vi "test_Set Slot.vi"(8 "error in (no error)":errorcluster, 11 "TestCase in":refnum<class "Scan Engine Scripting API Custom Device Unit Tests.lvclass">) -> (0 "error out":errorcluster, 3 "TestCase out":refnum<class "Scan Engine Scripting API Custom Device Unit Tests.lvclass">)   [LabVIEW 2020, in "Scan Engine Scripting API Custom Device Unit Tests.lvclass"]
uses:
  Scan Engine Scripting API Custom Device Unit Tests.lvclass
  Scan Engine Scripting API Custom Device Unit Tests.lvclass/Scan Engine Scripting API Custom Device Unit Tests.ctl
  Scripting/Modules/NI 9475/NI 9475.lvclass
  <vilib>/Addons/_JKI Toolkits/VI Tester/TestCase.llb/TestCase.lvclass
  Scripting/Scan Engine Scripting.lvlib
  Scripting/Modules/Mode Classes/Controls/digital channel settings.ctl
  C:/Users/Administrator/Desktop/Jatin/All DNC DLLs/NationalInstruments.VeriStand.SystemDefinitionAPI.dll
  Jatin/All DNC DLLs/NationalInstruments.VeriStand.SystemDefinitionAPI.dll
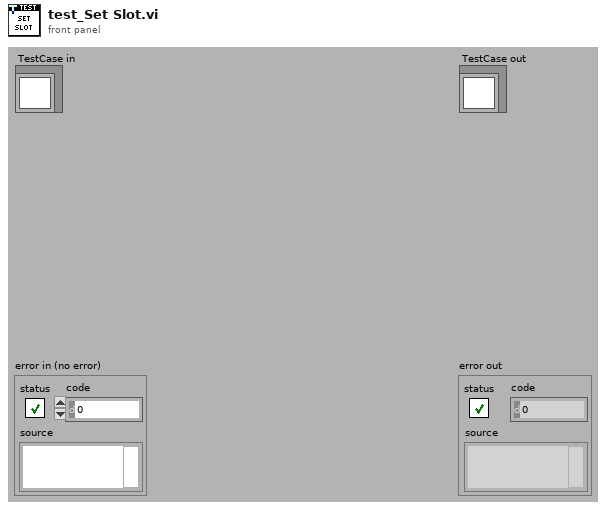
[diagram p1: front panel]
types:
  T1 = typedef "Scan Engine Scripting.lvlib/digital channel settings.ctl" = cluster{"name":string, "default value":bool}
  T2 = typedef "Custom Device API.lvlib/Custom Device Item Ref.ctl" = u64
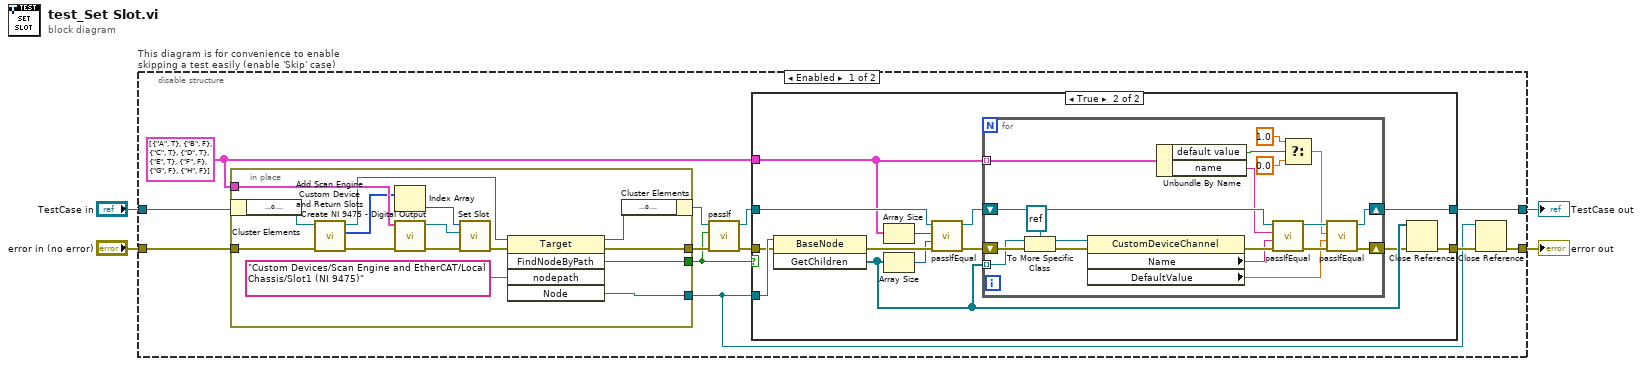
[diagram p0: block diagram]
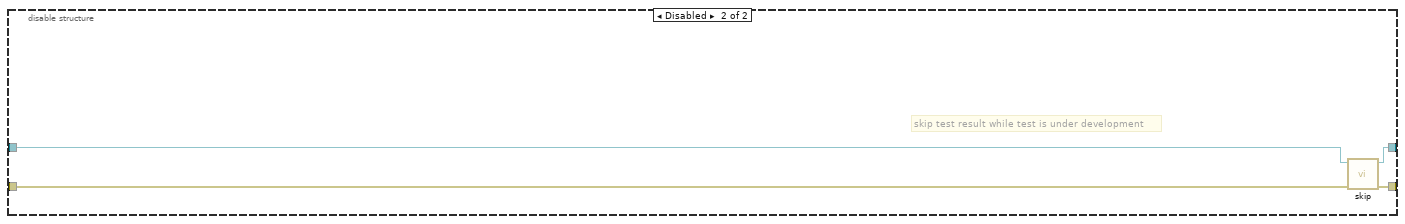
[diagram p3: hidden frame]
diagram:
  n1 = disable-structure "This diagram is for convenience to enable skipping a test easily (enable 'Skip' case)" shown="Enabled" {
    disable-tunnel: "TestCase in" -> [w8 w69]
    disable-tunnel: [w11 w67] -> w1
    disable-tunnel: [w10 w68] -> w3
    disable-tunnel: "error in (no error)" -> [w9 w66]
    frame Enabled {
      w6 = T1[] [{"name"="A", "default value"=TRUE}, {"name"="B", "default value"=FALSE}, {"name"="C", "default value"=TRUE}, {"name"="D", "default value"=TRUE}, {"name"="E", "default value"=TRUE}, {"name"="F", "default value"=FALSE}, {"name"="G", "default value"=FALSE}, {"name"="H", "default value"=FALSE}] ("channel settings")
      n2 = in-place {
        in-place-border: [w59] -> w16
        in-place-border: [w58] -> w5
        in-place-border: [w57] -> w15
        in-place-border: w9 -> [w55]
        in-place-border: w6 -> [w65]
        n3 = in-place-cluster #1(w8) -> ("target ref"=w52:refnum<k24>)
        n4 = call "Add Scan Engine Custom Device and Return Slots.vi"("error in"=w55, "NationalInstruments.VeriStand.SystemDefinitionAPI.Target"=w52) -> ("error out"=w54:errorcluster, "slot refs"=w53:T2[], "NationalInstruments.VeriStand.SystemDefinitionAPI.Target"=w56:refnum<k39>)  [unwired: 7 in]
        n5 = Index Array(array=w53) -> (element=w64:T2)  [unwired: 1 in]
        n6 = call "Create NI 9475 - Digital Output.vi"("error in"=w54, "channel settings"=w65) -> ("error out"=w63:errorcluster, "NI 9475 out"=w62:refnum<class "NI 9475.lvclass">)  [unwired: 8 in]
        n7 = call "Set Slot.vi"("error in"=w63, "module"=w62, "slot ref in"=w64) -> ("error out"=w61:errorcluster)  [unwired: 7 in, 1 out]
        n8 = invoke class="Target" method="FindNodeByPath"(reference=w56, error in=w61, "nodepath"="Custom Devices/Scan Engine and EtherCAT/Local Chassis/Slot1 (NI 9475)") -> (reference out=w51:refnum<k39>, error out=w59:errorcluster, "FindNodeByPath"=w57:bool, "Node"=w58:refnum<k39>)  [unwired: 2 in, 1 out]
        n9 = in-place-cluster #1("target ref"=w51) -> (w7:refnum<class "Scan Engine Scripting API Custom Device Unit Tests.lvclass">)
      }
      n10 = call-dynamic "passIf.vi"("error in (no error)"=w16, "pass"=w15, "TestCase in"=w7) -> ("error out"=w13:errorcluster, "TestCase out"=w14:refnum<class "Scan Engine Scripting API Custom Device Unit Tests.lvclass">)  [unwired: 7 in]
      n11 = case shown="True" w15 {
        tunnel: w13 -> [w17 w30]
        tunnel: w14 -> [w18 w29]
        tunnel: w5 -> [_ w31]
        tunnel: [w18 w22] -> w11
        tunnel: [w17 w27] -> w12
        tunnel: w6 -> [_ w21]
        frame False {
        }
        frame True {
          n12 = invoke class="BaseNode" method="GetChildren"(reference=w31, error in=w30) -> (error out=w28:errorcluster, "GetChildren"=w26:refnum<k39>[])  [unwired: 1 in, 1 out]
          n13 = Array Size(array=w21) -> (size(s)=w20:i32)
          n14 = Array Size(array=w26) -> (size(s)=w19:i32)
          n15 = call-dynamic "passIfEqual.vi"("error in (no error)"=w28, "y"=w19, "x"=w20, "TestCase in"=w29) -> ("error out"=w25:errorcluster, "TestCase out"=w23:refnum<class "Scan Engine Scripting API Custom Device Unit Tests.lvclass">)  [unwired: 6 in]
          n16 = for {
            tunnel: w26 -> [w32] mode=indexing
            shift-right: [w38] -> w24
            shift-left: w25 -> [w49]
            tunnel: w21 -> [w37] mode=indexing
            shift-right: [w39] -> w22
            shift-left: w23 -> [w40]
            n17 = To More Specific Class(target class=refnum<k39> refnum, reference=w32, error in=w49) -> (specific class reference=w48:refnum<k39>, error out=w47:errorcluster)
            n18 = property class="CustomDeviceChannel"(reference=w48, error in=w47) -> (error out=w46:errorcluster, "Name"=w34:string, "DefaultValue"=w36:dbl)  [unwired: 1 out]
            n19 = Unbundle By Name(w37) -> ("default value"=w45:bool, "name"=w33:string)
            n20 = call-dynamic "passIfEqual.vi"("error in (no error)"=w46, "y"=w34, "x"=w33, "TestCase in"=w40) -> ("error out"=w42:errorcluster, "TestCase out"=w41:refnum<class "Scan Engine Scripting API Custom Device Unit Tests.lvclass">)  [unwired: 6 in]
            n21 = Select(t=1.0, s=w45, f=0.0) -> (s? t:f=w35:dbl)
            n22 = call-dynamic "passIfEqual.vi"("error in (no error)"=w42, "y"=w36, "x"=w35, "TestCase in"=w41) -> ("error out"=w38:errorcluster, "TestCase out"=w39:refnum<class "Scan Engine Scripting API Custom Device Unit Tests.lvclass">)  [unwired: 6 in]
          }
          n23 = Close Reference(reference=w26, error in (no error)=w24) -> (error out=w27:errorcluster)
        }
      }
      n24 = Close Reference(reference=w5, error in (no error)=w12) -> (error out=w10:errorcluster)
    }
    frame Disabled {
      # "skip test result while test is under development"
      n25 = call <vilib>:"skip.vi"("error in (no error)"=w66, "TestCase in"=w69) -> ("error out"=w68:errorcluster, "TestCase out"=w67:refnum<class "Scan Engine Scripting API Custom Device Unit Tests.lvclass">)  [unwired: 8 in]
    }
  }
  "error out" <- w3
  "TestCase out" <- w1
